vi "1.vi"(9 "Numeric":i32, 10 "1":dbl, 11 "Numeric 2":i32) -> (3 "Array":u32[](array[numeric]))   [LabVIEW 2016]
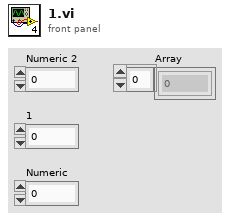
[diagram p1: front panel]
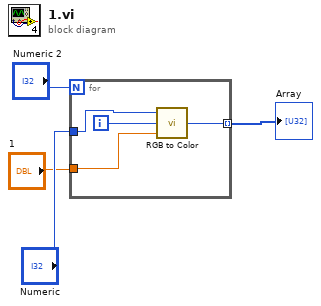
[diagram p0: block diagram]
diagram:
  n1 = for {
    N: "Numeric 2" -> [_]
    tunnel: [w8] -> w1 mode=indexing
    tunnel: "Numeric" -> [w5]
    tunnel: "1" -> [w7]
    i -> [w6]
    n2 = call <vilib>:"RGB to Color.vi"("B"=w7, "G"=w6, "R"=w5) -> ("Color"=w8:u32)
  }
  "Array" <- w1
